vi "test1.vi"() -> ()   [LabVIEW 2018]
uses:
  src/TcpServer/TcpServer.lvclass
  src/TcpServer/runServer.vi
  src/TcpServer/configServerTypeDef.ctl
  src/TcpServerTel/typedef/enqueueOptionsTypeDef.ctl
  src/TcpServerTel/TcpServerTel.lvclass
panel:
  out "connStatusMsg":string
  out "tcpPacket":string
  out "Clients Connected":bool
  out "error out":errorcluster
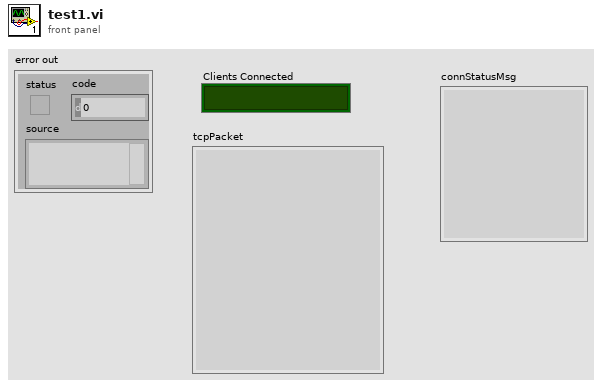
[diagram p1: front panel]
types:
  T1 = typedef "TcpServer.lvclass/configServerTypeDef.ctl" = cluster{"cmdServerPort":u16, "telServerPort":u16, "timeoutServerInMs":i32, "serverBytesToRead":i32, "maxSizeQueueTcpClientFromDds":i32, "EnqueueOptions":T2, "timeoutQueueTcpClientFromDds (ms)":i32, "maxSizeQueueTcpClient":i32, "timeoutInMs":i32}
  T2 = typedef "TcpServerTel.lvclass/enqueueOptionsTypeDef.ctl" = enum16{"lossy enqueue", "normal enqueue"}
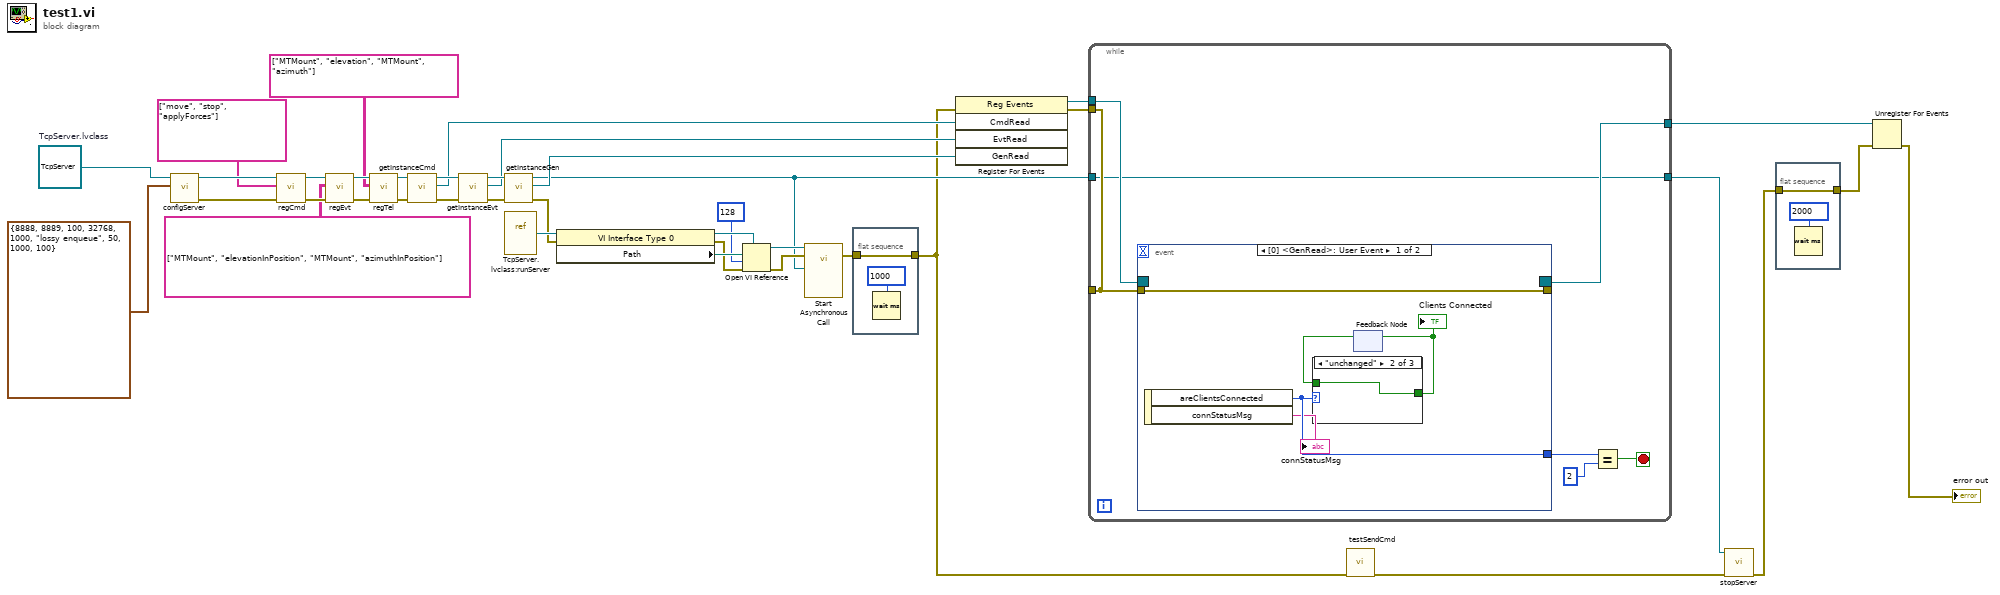
[diagram p0: block diagram]
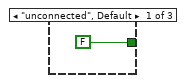
[diagram p2: hidden frame]
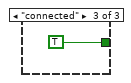
[diagram p3: hidden frame]
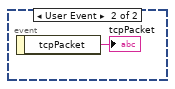
[diagram p4: hidden frame]
diagram:
  w39 = refnum<class "TcpServer.lvclass"> refnum  # TcpServer.lvclass
  n1 = call "configServer.vi"("ServerConfiguration"=T1 {"cmdServerPort"=8888, "telServerPort"=8889, "timeoutServerInMs"=100, "serverBytesToRead"=32768, "maxSizeQueueTcpClientFromDds"=1000, "EnqueueOptions"=enum."lossy enqueue", "timeoutQueueTcpClientFromDds (ms)"=50, "maxSizeQueueTcpClient"=1000, "timeoutInMs"=100}, "tcpServer in"=w39) -> ("error out"=w17:errorcluster, "tcpServer out"=w37:refnum<class "TcpServer.lvclass">)  [unwired: 8 in]
  n2 = call "regCmd.vi"("error in (no error)"=w17, "cmdReg"=string[] ["move", "stop", "applyForces"], "tcpServer in"=w37) -> ("error out"=w38:errorcluster, "tcpServer out"=w24:refnum<class "TcpServer.lvclass">)  [unwired: 7 in]
  n3 = call "regEvt.vi"("error in (no error)"=w38, "evtReg"=string[][] [["MTMount", "elevationInPosition"], ["MTMount", "azimuthInPosition"]], "tcpServer in"=w24) -> ("error out"=w25:errorcluster, "tcpServer out"=w20:refnum<class "TcpServer.lvclass">)  [unwired: 7 in]
  n4 = call "regTel.vi"("error in (no error)"=w25, "telReg"=string[][] [["MTMount", "elevation"], ["MTMount", "azimuth"]] ("regTel"), "tcpServer in"=w20) -> ("error out"=w21:errorcluster, "tcpServer out"=w19:refnum<class "TcpServer.lvclass">)  [unwired: 7 in]
  n5 = call "getInstanceCmd.vi"("error in (no error)"=w21, "tcpServer in"=w19) -> ("error out"=w36:errorcluster, "CmdRead"=w13:refnum<user-event>, "tcpServer out"=w34:refnum<class "TcpServer.lvclass">)  [unwired: 7 in]
  n6 = call "getInstanceEvt.vi"("error in (no error)"=w36, "tcpServer in"=w34) -> ("error out"=w35:errorcluster, "EvtRead"=w12:refnum<user-event>, "tcpServer out"=w22:refnum<class "TcpServer.lvclass">)  [unwired: 7 in]
  n7 = call "getInstanceGen.vi"("error in (no error)"=w35, "tcpServer in"=w22) -> ("error out"=w23:errorcluster, "GenRead"=w11:refnum<user-event>, "tcpServer out"=w6:refnum<class "TcpServer.lvclass">)  [unwired: 7 in]
  n8 = vi-ref "TcpServer.lvclass:runServer.vi"() -> (w33:refnum<vi>)
  n9 = property class="VI Interface Type 0"(reference=w33, error in=w23) -> (reference out=w31:refnum<vi>, error out=w28:errorcluster, "Path"=w32:path)
  n10 = Open VI Reference(type specifier VI Refnum (for type only)=w31, vi path=w32, options=128, error in (no error)=w28) -> (vi reference=w29:refnum<vi>, error out=w27:errorcluster)  [unwired: 2 in]
  n11 = call-by-ref "Start Asynchronous Call"(reference=w29, error in=w27, "TcpServer in"=w6) -> (error out=w26:errorcluster)  [unwired: 9 in, 3 out]
  n12 = flat-sequence {
    tunnel: w26 -> [w40]
    tunnel: [w40] -> w3
    frame #0 {
      n13 = Wait (ms)(milliseconds to wait=u32 1000) -> ()  [unwired: 1 out]
    }
  }
  n14 = register-events(error in=w3, w13, w12, w11) -> (reference out=w9:refnum<event-registration>, error out=w10:errorcluster)  [unwired: 1 in]
  n15 = while {
    tunnel: [w48] -> _
    tunnel: w10 -> [w48]
    tunnel: w9 -> [w47]
    tunnel: [w46] -> w8
    tunnel: [w45] -> w7
    tunnel: w6 -> [w45]
    stop <- w42 stop-if-true
    n16 = event shown="[0] <GenRead>: User Event" {
      selector: w47 -> [_ _]
      dyn-events: [_ _] -> w46
      timeout: _ -> [_ _]
      tunnel: [w53 _] -> _
      tunnel: w48 -> [w53 _]
      tunnel: [w50 _] -> w44
      event User Event {
        n17 = event-data() -> ("areClientsConnected"=w50:enum16{"unchanged", "connected", "unconnected"}, "connStatusMsg"=→"connStatusMsg":string)  [unwired: 1 in]
        n18 = feedback #1() -> (w52:bool)  [unwired: 1 in]
        n19 = case shown="\"unchanged\"" w50 {
          tunnel: [FALSE w55 TRUE] -> w51
          tunnel: w52 -> [_ w55 _]
          frame "unconnected", Default {
          }
          frame "unchanged" {
          }
          frame "connected" {
          }
        }
        "Clients Connected" <- w51
        n20 = feedback-in #1(w51) -> ()
      }
      event User Event {
        n21 = event-data() -> ("tcpPacket"=→"tcpPacket":string)  [unwired: 1 in]
      }
    }
    n22 = Equal?(x=w44, y=2) -> (x = y?=w42:bool)
  }
  n23 = call "testSendCmd.vi"("error in (no error)"=w3) -> ("error out"=w4:errorcluster)  [unwired: 10 in]
  n24 = call "stopServer.vi"("error in (no error)"=w4, "tcpServer in"=w7) -> ("error out"=w2:errorcluster)  [unwired: 8 in, 1 out]
  n25 = flat-sequence {
    tunnel: w2 -> [w58]
    tunnel: [w58] -> w1
    frame #0 {
      n26 = Wait (ms)(milliseconds to wait=u32 2000) -> ()  [unwired: 1 out]
    }
  }
  n27 = Unregister For Events(event registration refnum=w8, error in=w1) -> (error out=→"error out":errorcluster)
